vi "app-dir_to_server-dir.vi"(11 "Application Directory":string) -> (3 "Group Server Directory":string)   [LabVIEW 2016]
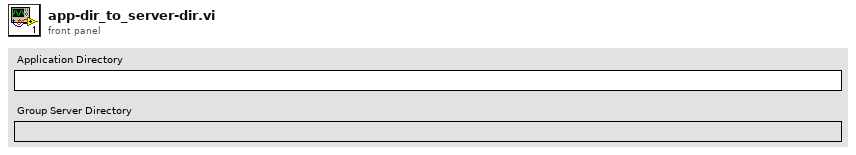
[diagram p1: front panel]
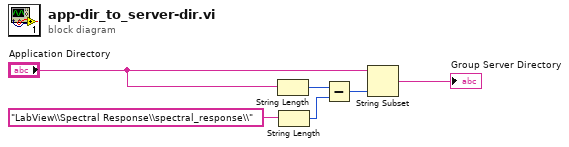
[diagram p0: block diagram]
diagram:
  n1 = String Length(string="Application Directory") -> (length=w3:i32)
  n2 = String Length(string="LabView\\Spectral Response\\spectral_response\\" ("regular expression")) -> (length=w2:i32)
  n3 = Subtract(x=w3, y=w2) -> (x-y=w1:i32)
  n4 = String Subset(string="Application Directory", length (rest)=w1) -> (substring=→"Group Server Directory":string)  [unwired: 1 in]
